vi "Write Amplitude Test Values.vi"(10 "Test Values":T1 {"Stop Value" format="%.3f"; "Start Value" format="%.3f"}, 11 "Model in":refnum<class "Model.lvclass">) -> (3 "Model out":refnum<class "Model.lvclass">)   [LabVIEW 2015]
uses:
  Model.lvclass
  Typedefs/Test Values.ctl
  Typedefs/FAMTTypedefs.lvlib
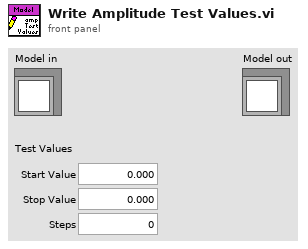
[diagram p1: front panel]
types:
  T1 = typedef "FAMTTypedefs.lvlib/Test Values.ctl" = cluster{"Start Value":dbl, "Stop Value":dbl, "Steps":u16}
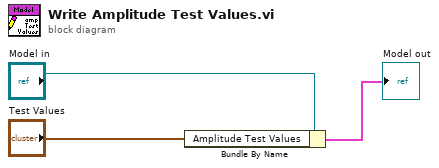
[diagram p0: block diagram]
diagram:
  n1 = Bundle By Name(cluster="Model in", "Amplitude Test Values"="Test Values") -> (→"Model out":cluster{})
